vi "Controller Apply Configuration from GUI.vi"(7 "Sync Objects":T9, 8 "error in (no error)":errorcluster, 10 "Configuration Data (GUI to Controller)":T8, 11 "FOFB Configuration":T1={"FOFB Parameters"={"Network"={"FOFB Controller IP"="", "LNLS Control Network IP"="", "LNLS Control Network Power Supplies TCP Port"=0, "LNLS Control Network FOFB Configuration TCP Port"=0, "LNLS Control Network BPMs TCP Port"=0, "Data Server TCP Port"=0, "Monitoring Data TCP Port"=0, "Configuration GUI TCP Port"=0, "Storage Data TCP Port"=0, "Fast Command TCP Port"=0, "TCP Listening Timeout"=0}, "Fast Acquisition"={"Sampling Period"=0, "Data Buffer Size"=0, "Monitoring Period"=0}, "Acquisition Network"=[], "Actuation Network"=[]}, "Number of Acquisition Chassis"=0, "Number of Actuation Chassis"=0, "Number of BPM Readings"=0, "BPM Reading Names"=[], "Selected BPM Readings"=[0, 1, 2, 3, 4, 5, 6, 7, 8, 9, 10, 11, 12, 13, 14, 15, 16, 17, 18, 19, 20, 21, 22, 23, 24, 25, 26, 27, 28, 29, 30, 31, 32, 33, 34, 35, 36, 37, 38, 39, 40, 41, 42, 43, 44, 45, 46, 47, 48, 49], "Number of Correctors"=0, "Corrector Names"=[], "Selected Correctors"=[0, 1, 2, 3, 4, 5, 6, 7, 8, 9, 10, 11, 12, 13, 14, 15, 16, 17, 18, 19, 20, 21, 22, 23, 24, 25, 26, 27, 28, 29, 30, 31, 32, 33, 34, 35, 36, 37, 38, 39, 40, 41, 42, 43, 44, 45, 46, 47, 48, 49], "Reference Orbit"=[], "Response Matrix"=[], "Correction Matrix"=[], "Acquisition Chassis Names"=[], "Actuation Chassis Names"=[], "Acquisition Variables"=[], "Actuation Variables"=[], "PS Matrix Mapping"=[], "Inverse PS Matrix Mapping"=[], "BPM Matrix Mapping"=[], "Inverse BPM Matrix Mapping"=[], "BPM Planes"=[], "Corrector Planes"=[]}) -> (0 "error out":errorcluster, 2 "Configuration Change Acknowledge (Controller to GUI)":T7)   [LabVIEW 2011, in "Controller VIs.lvlib"]
uses:
  Controller VIs.lvlib
  Types Definitions/Type Synchronization Objects.ctl
  Types Definitions/Type Blocking Synchronization Objects.ctl
  Types Definitions/Type Monitoring Data.ctl
  Types Definitions/Type Operation Mode State.ctl
  Types Definitions/Type Diagnostics Data.ctl
  Types Definitions/Type CPU Loads Array.ctl
  Types Definitions/Type CPU Loads.ctl
  Types Definitions/Type Non-blocking Synchronization Objects.ctl
  Types Definitions/Type FOFB Variables.ctl
  Types Definitions/Type Actuation State.ctl
  Types Definitions/Type Configuration Data (GUI to Controller).ctl
  Types Definitions/Type FOFB Parameters.ctl
  Types Definitions/Type Network Configuration.ctl
  Types Definitions/Type FA Configuration.ctl
  Types Definitions/Type Acquisition Network Configuration.ctl
  Types Definitions/Type Actuation Network Configuration.ctl
  Types Definitions/Type Configuration Change Acknowledge (Controller to GUI).ctl
  Types Definitions/Type FOFB Configuration.ctl
  File VIs/File Read Orbit.vi
  File VIs/File Read Matrix.vi
  XML VIs/XML Get Actuation Chassis.vi
  XML VIs/XML Get Acquisition Chassis.vi
  Controller Orbit Correction Matrix Calculation.vi
  File VIs/File Write Matrix.vi
  Type Definitions.lvlib
  XML VIs.lvlib
  File VIs.lvlib
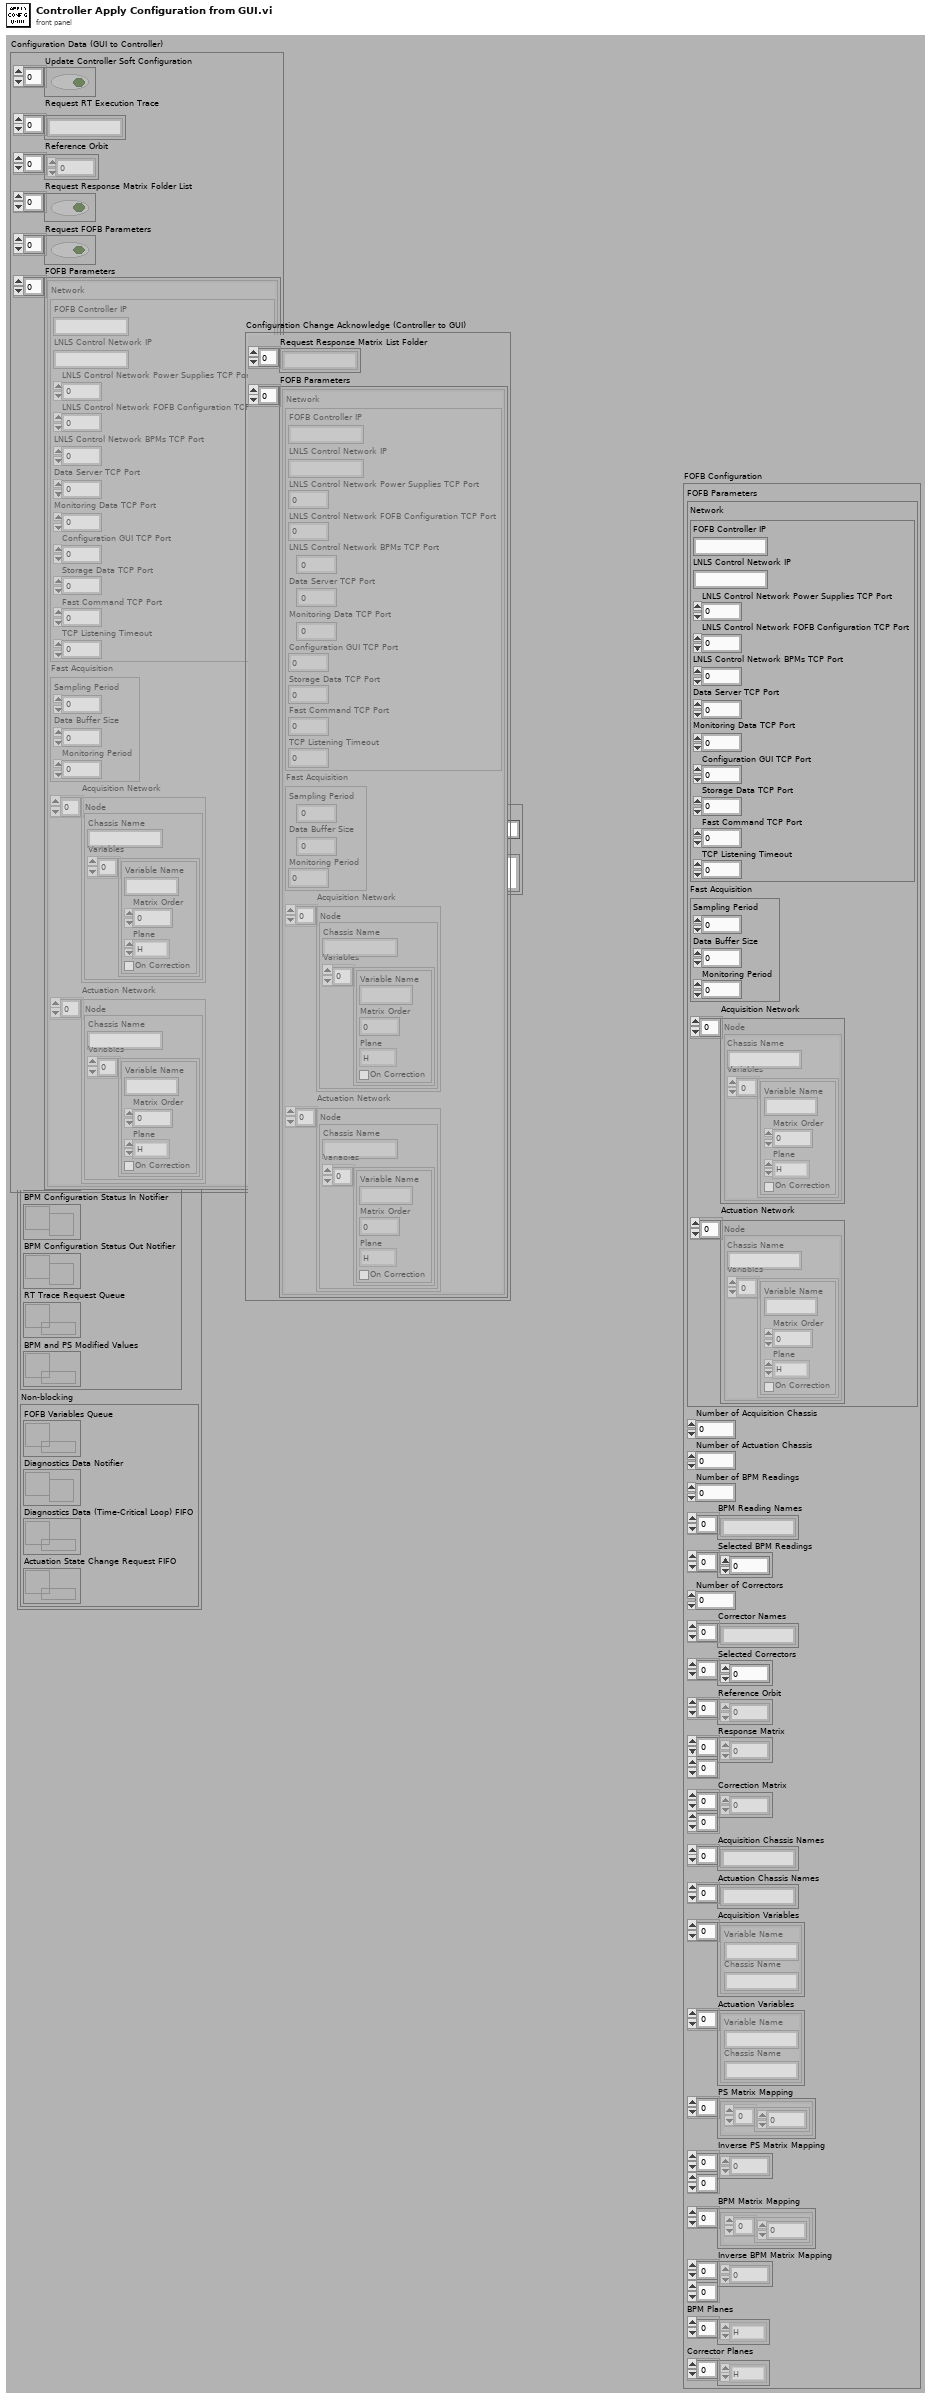
[diagram p1: front panel]
types:
  T1 = typedef "Type Definitions.lvlib/Type FOFB Configuration.ctl" = cluster{"FOFB Parameters":T2, "Number of Acquisition Chassis":i32, "Number of Actuation Chassis":i32, "Number of BPM Readings":i32, "BPM Reading Names":string[], "Selected BPM Readings":u32[], "Number of Correctors":i32, "Corrector Names":string[], "Selected Correctors":u32[], "Reference Orbit":dbl[], "Response Matrix":dbl[][], "Correction Matrix":dbl[][], "Acquisition Chassis Names":string[], "Actuation Chassis Names":string[], "Acquisition Variables":cluster{"Variable Name":string, "Chassis Name":string}[], "Actuation Variables":cluster{"Variable Name":string, "Chassis Name":string}[], "PS Matrix Mapping":cluster{u32[]}[], "Inverse PS Matrix Mapping":u32[][], "BPM Matrix Mapping":cluster{u32[]}[], "Inverse BPM Matrix Mapping":u32[][], "BPM Planes":enum8{"H", "V"}[], "Corrector Planes":enum8{"H", "V"}[]}
  T2 = typedef "Type Definitions.lvlib/Type FOFB Parameters.ctl" = cluster{"Network":T3, "Fast Acquisition":T4, "Acquisition Network":T5, "Actuation Network":T6}
  T3 = typedef "Type Definitions.lvlib/Type Network Configuration.ctl" = cluster{"FOFB Controller IP":string, "LNLS Control Network IP":string, "LNLS Control Network Power Supplies TCP Port":u16, "LNLS Control Network FOFB Configuration TCP Port":u16, "LNLS Control Network BPMs TCP Port":u16, "Data Server TCP Port":u16, "Monitoring Data TCP Port":u16, "Configuration GUI TCP Port":u16, "Storage Data TCP Port":u16, "Fast Command TCP Port":u16, "TCP Listening Timeout":i32}
  T4 = typedef "Type Definitions.lvlib/Type FA Configuration.ctl" = cluster{"Sampling Period":u32, "Data Buffer Size":u32, "Monitoring Period":u32}
  T5 = typedef "Type Definitions.lvlib/Type Acquisition Network Configuration.ctl" = cluster{"Chassis Name":string, "Variables":cluster{"Variable Name":string, "Matrix Order":u32, "Plane":enum8{"H", "V"}, "On Correction":bool}[]}[]
  T6 = typedef "Type Definitions.lvlib/Type Actuation Network Configuration.ctl" = cluster{"Chassis Name":string, "Variables":cluster{"Variable Name":string, "Matrix Order":u32, "Plane":enum8{"H", "V"}, "On Correction":bool}[]}[]
  T7 = typedef "Type Definitions.lvlib/Type Configuration Change Acknowledge (Controller to GUI).ctl" = cluster{"Request Response Matrix List Folder":string[], "FOFB Parameters":T2[]}
  T8 = typedef "Type Definitions.lvlib/Type Configuration Data (GUI to Controller).ctl" = cluster{"Update Controller Soft Configuration":bool[], "Request RT Execution Trace":string[], "Reference Orbit":dbl[], "Request Response Matrix Folder List":bool[], "Request FOFB Parameters":bool[], "FOFB Parameters":T2[]}
  T9 = typedef "Type Definitions.lvlib/Type Synchronization Objects.ctl" = cluster{"Blocking":T10, "Non-blocking":T11}
  T10 = typedef "Type Definitions.lvlib/Type Blocking Synchronization Objects.ctl" = cluster{"Monitoring Data Notifier":refnum<notifier>, "Storage Data FIFO":refnum<queue>, "Operation Mode Change Request FIFO":refnum<k33>, "Monitoring BPM and PS Data FIFO":refnum<k33>, "FA BPM and PS Data FIFO":refnum<k33>, "PS Manual Setpoints FIFO":refnum<k33>, "FOFB Controller Errors FIFO ":refnum<k33>, "FOFB Status In Notifier":refnum<notifier>, "FOFB Status Out Notifier":refnum<notifier>, "PS Configuration Status In Notifier":refnum<notifier>, "PS Configuration Status Out Notifier":refnum<notifier>, "BPM Configuration Status In Notifier":refnum<notifier>, "BPM Configuration Status Out Notifier":refnum<notifier>, "RT Trace Request Queue":refnum<queue>, "BPM and PS Modified Values":refnum<k33>}
  T11 = typedef "Type Definitions.lvlib/Type Non-blocking Synchronization Objects.ctl" = cluster{"FOFB Variables Queue":refnum<queue>, "Diagnostics Data Notifier":refnum<notifier>, "Diagnostics Data (Time-Critical Loop) FIFO":refnum<k33>, "Actuation State Change Request FIFO":refnum<k33>}
  T12 = typedef "Type Definitions.lvlib/Type FOFB Variables.ctl" = cluster{"Reference Orbit":dbl[], "Response Matrix":dbl[][], "Correction Matrix":dbl[][], "Selected BPM Readings":u32[], "Selected Correctors":u32[], "BPM Planes":enum8{"H", "V"}[], "Corrector Planes":enum8{"H", "V"}[], "Fast Command Enabled":bool, "Horizontal Gain":dbl, "Vertical Gain":dbl}
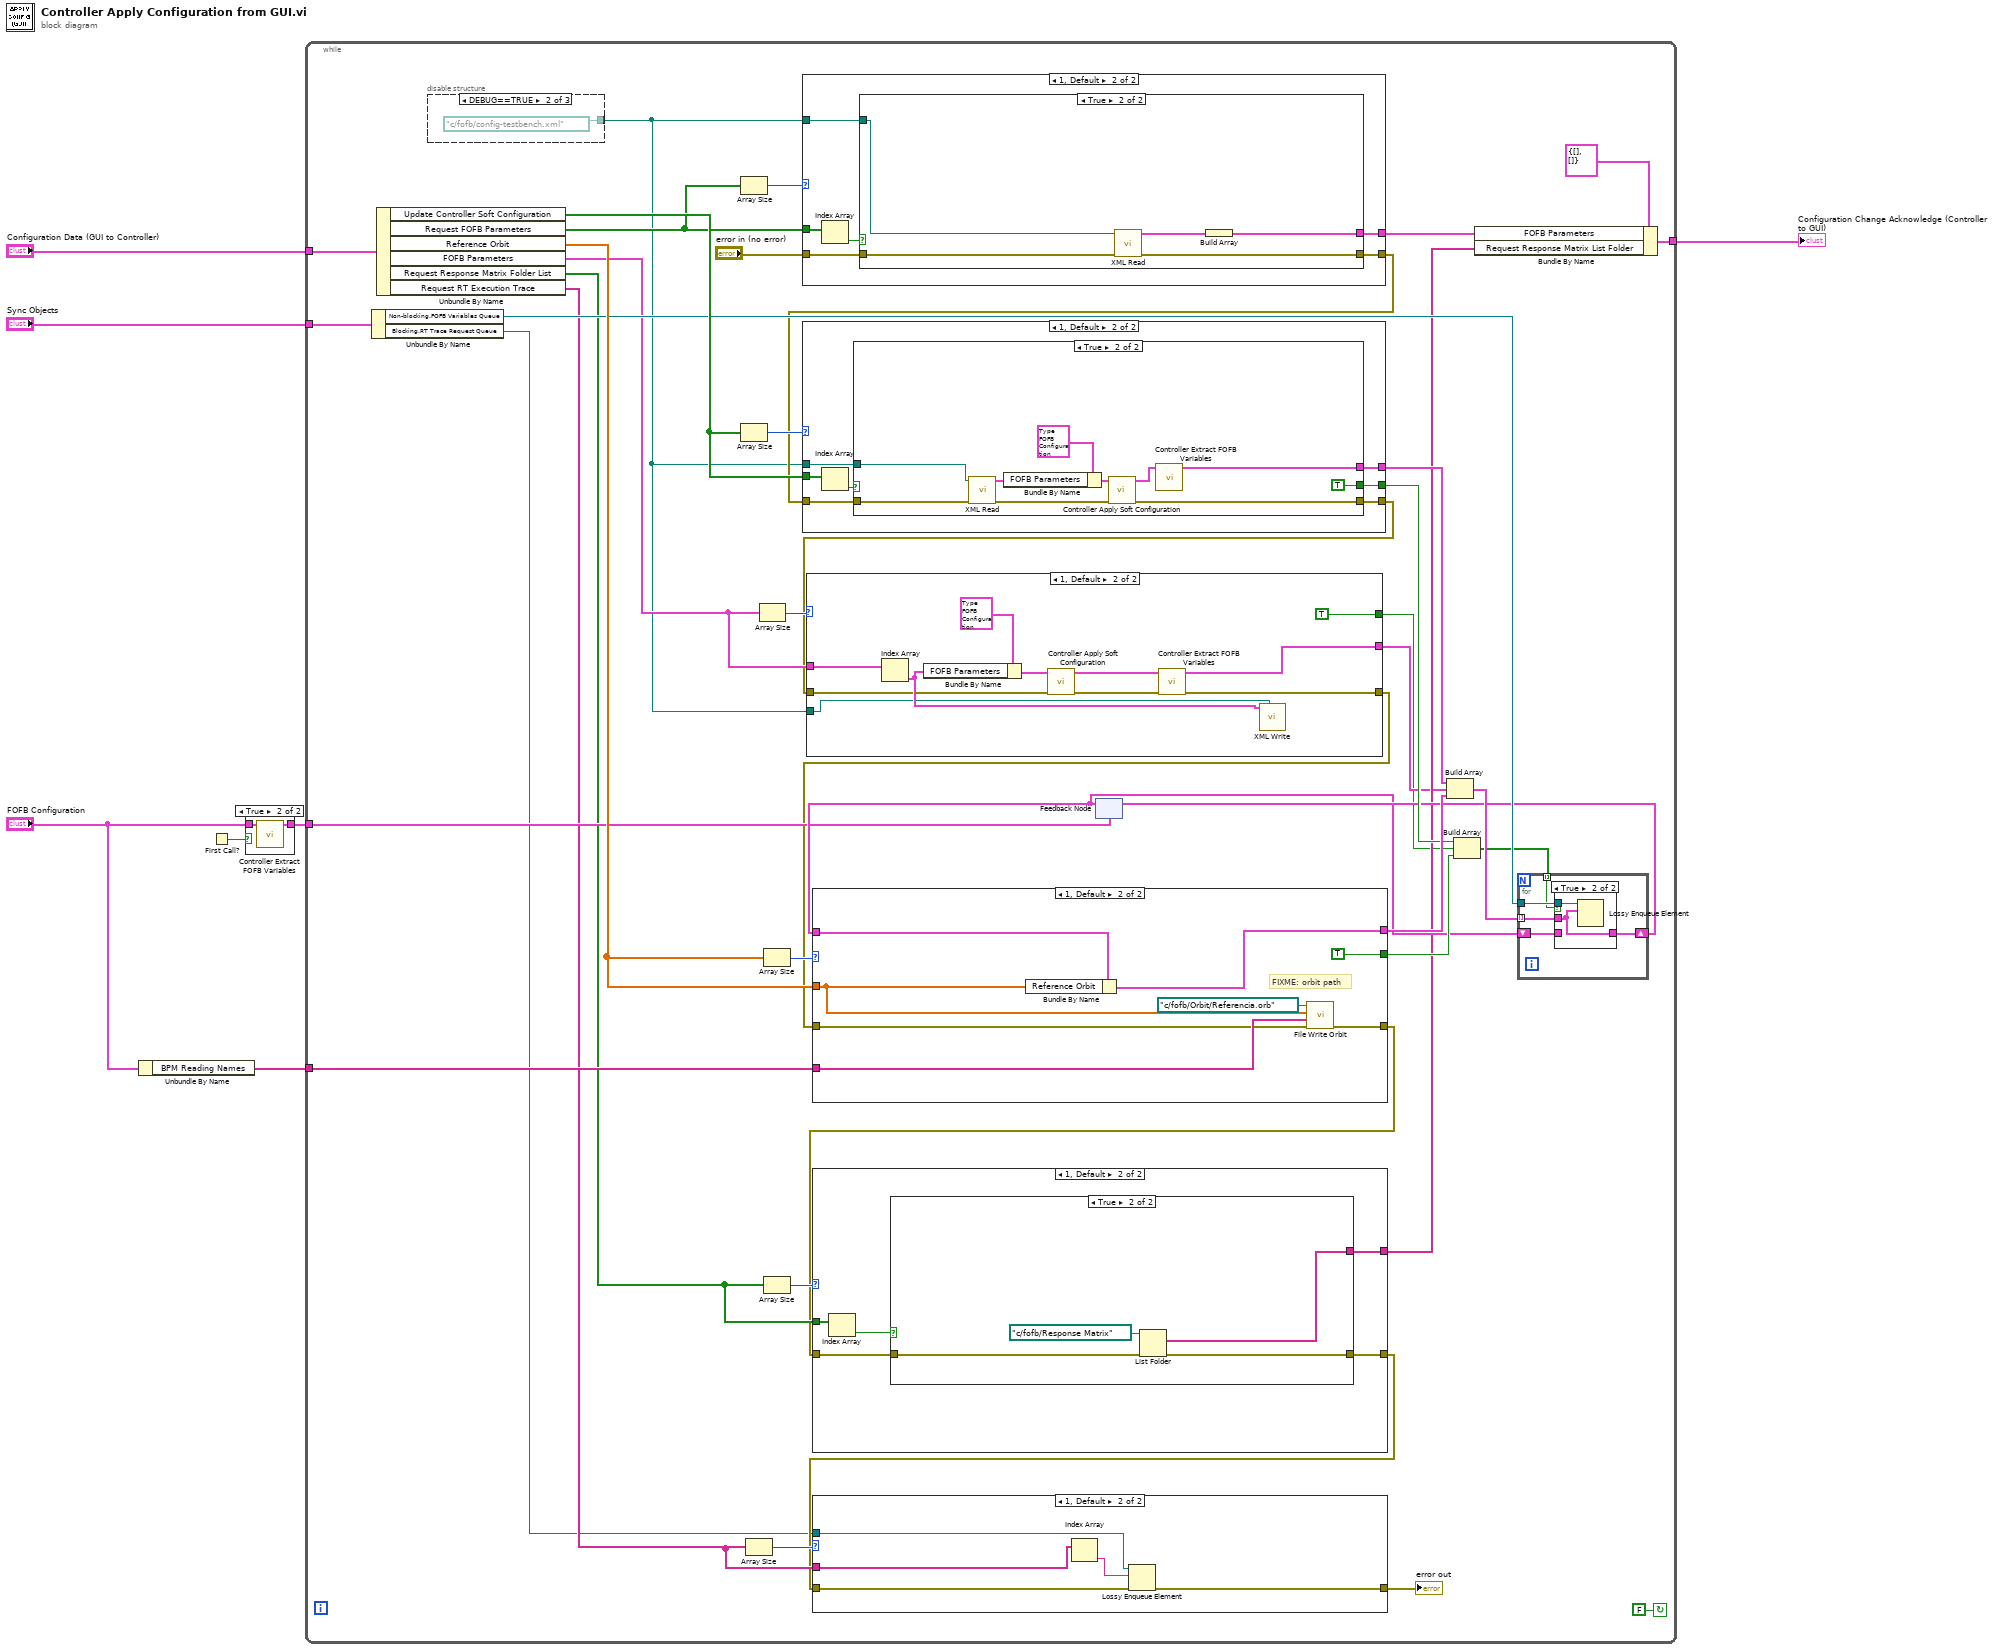
[diagram p0: block diagram]
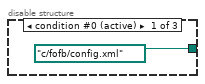
[diagram p4: hidden frame]
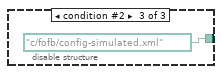
[diagram p5: hidden frame]
diagram:
  n1 = Unbundle By Name("FOFB Configuration") -> ("BPM Reading Names"=w1:string[])
  n2 = First Call?() -> (First Call?: T/F=w4:bool)
  n3 = case shown="True" w4 {
    tunnel: "FOFB Configuration" -> [_ w9]
    tunnel: [_ w8] -> w3
    frame False {
    }
    frame True {
      n4 = call "Controller Extract FOFB Variables.vi"("FOFB Configuration"=w9) -> ("FOFB Variables"=w8:T12)  [unwired: 9 in, 1 out]
    }
  }
  n5 = while {
    tunnel: "Sync Objects" -> [w50]
    tunnel: "Configuration Data (GUI to Controller)" -> [w49]
    tunnel: [w40] -> w5
    tunnel: w3 -> [w28]
    tunnel: w1 -> [w27]
    stop <- FALSE continue-if-true
    n6 = Unbundle By Name(w50) -> ("Non-blocking.FOFB Variables Queue"=w39:refnum<queue>, "Blocking.RT Trace Request Queue"=w17:refnum<queue>)
    n7 = Unbundle By Name(w49) -> ("Update Controller Soft Configuration"=w46:bool[], "Request FOFB Parameters"=w44:bool[], "Reference Orbit"=w41:dbl[], "FOFB Parameters"=w15:T2[], "Request Response Matrix Folder List"=w25:bool[], "Request RT Execution Trace"=w20:string[])
    n8 = disable-structure shown="DEBUG==TRUE" {
      disable-tunnel: [path "c:/fofb/config.xml" ("Configuration File Path") path "c:/fofb/config-testbench.xml" ("Configuration File Path") path "c:/fofb/config-simulated.xml" ("Configuration File Path")] -> w13
      frame condition #0 (active) {
      }
      frame condition #1 {
      }
      frame condition #2 {
      }
    }
    n9 = Array Size(array=w44) -> (size(s)=w45:i32)
    n10 = Array Size(array=w46) -> (size(s)=w47:i32)
    n11 = Array Size(array=w20) -> (size(s)=w21:i32)
    n12 = Array Size(array=w15) -> (size(s)=w16:i32)
    n13 = Array Size(array=w41) -> (size(s)=w42:i32)
    n14 = Array Size(array=w25) -> (size(s)=w26:i32)
    n15 = case shown="1, Default" w45 {
      tunnel: w44 -> [_ w107]
      tunnel: "error in (no error)" -> [w101 w105]
      tunnel: [w101 w104] -> w38
      tunnel: [_ w103] -> w43
      tunnel: w13 -> [_ w102]
      frame 0 {
      }
      frame 1, Default {
        n16 = Index Array(array=w107) -> (element=w106:bool)  [unwired: 1 in]
        n17 = case shown="True" w106 {
          tunnel: w105 -> [w108 w113]
          tunnel: [w108 w112] -> w104
          tunnel: [_ w111] -> w103
          tunnel: w102 -> [_ w109]
          frame False {
          }
          frame True {
            n18 = call "XML Read.vi"("error in"=w113, "XML File Path In"=w109) -> ("error out"=w112:errorcluster, "FOFB Parameters"=w110:T2)  [unwired: 8 in]
            n19 = Build Array(w110) -> (w111:T2[])
          }
        }
      }
    }
    n20 = case shown="1, Default" w47 {
      tunnel: w46 -> [_ w121]
      tunnel: w38 -> [w114 w119]
      tunnel: [w114 w117] -> w11
      tunnel: [_ w118] -> w37
      tunnel: [_ w116] -> w35
      tunnel: w13 -> [_ w115]
      frame 0 {
      }
      frame 1, Default {
        n21 = Index Array(array=w121) -> (element=w120:bool)  [unwired: 1 in]
        n22 = case shown="True" w120 {
          tunnel: w119 -> [w122 w129]
          tunnel: [w122 w126] -> w117
          tunnel: [_ w125] -> w118
          tunnel: [_ TRUE] -> w116
          tunnel: w115 -> [_ w123]
          frame False {
          }
          frame True {
            n23 = call "XML Read.vi"("error in"=w129, "XML File Path In"=w123) -> ("error out"=w132:errorcluster, "FOFB Parameters"=w130:T2)  [unwired: 8 in]
            n24 = Bundle By Name(cluster=T1 {"FOFB Parameters"={"Network"={"FOFB Controller IP"="", "LNLS Control Network IP"="", "LNLS Control Network Power Supplies TCP Port"=0, "LNLS Control Network FOFB Configuration TCP Port"=0, "LNLS Control Network BPMs TCP Port"=0, "Data Server TCP Port"=0, "Monitoring Data TCP Port"=0, "Configuration GUI TCP Port"=0, "Storage Data TCP Port"=0, "Fast Command TCP Port"=0, "TCP Listening Timeout"=0}, "Fast Acquisition"={"Sampling Period"=0, "Data Buffer Size"=0, "Monitoring Period"=0}, "Acquisition Network"=[], "Actuation Network"=[]}, "Number of Acquisition Chassis"=0, "Number of Actuation Chassis"=0, "Number of BPM Readings"=0, "BPM Reading Names"=[], "Selected BPM Readings"=[], "Number of Correctors"=0, "Corrector Names"=[], "Selected Correctors"=[], "Reference Orbit"=[], "Response Matrix"=[], "Correction Matrix"=[], "Acquisition Chassis Names"=[], "Actuation Chassis Names"=[], "Acquisition Variables"=[], "Actuation Variables"=[], "PS Matrix Mapping"=[], "Inverse PS Matrix Mapping"=[], "BPM Matrix Mapping"=[], "Inverse BPM Matrix Mapping"=[], "BPM Planes"=[], "Corrector Planes"=[]}, "FOFB Parameters"=w130) -> (w131:T1)
            n25 = call "Controller Apply Soft Configuration.vi"("error in (no error)"=w132, "FOFB Configuration"=w131) -> ("error out"=w126:errorcluster, "FOFB Configuration"=w128:T1)  [unwired: 8 in]
            n26 = call "Controller Extract FOFB Variables.vi"("FOFB Configuration"=w128) -> ("FOFB Variables"=w125:T12)  [unwired: 9 in, 1 out]
          }
        }
      }
    }
    n27 = case shown="1, Default" w16 {
      tunnel: w15 -> [_ w62]
      tunnel: [_ w58] -> w14
      tunnel: w13 -> [_ w56]
      tunnel: [_ TRUE] -> w12
      tunnel: w11 -> [w51 w54]
      tunnel: [w51 w52] -> w10
      frame 0 {
      }
      frame 1, Default {
        n28 = Index Array(array=w62) -> (element=w57:T2)  [unwired: 1 in]
        n29 = Bundle By Name(cluster=T1 {"FOFB Parameters"={"Network"={"FOFB Controller IP"="", "LNLS Control Network IP"="", "LNLS Control Network Power Supplies TCP Port"=0, "LNLS Control Network FOFB Configuration TCP Port"=0, "LNLS Control Network BPMs TCP Port"=0, "Data Server TCP Port"=0, "Monitoring Data TCP Port"=0, "Configuration GUI TCP Port"=0, "Storage Data TCP Port"=0, "Fast Command TCP Port"=0, "TCP Listening Timeout"=0}, "Fast Acquisition"={"Sampling Period"=0, "Data Buffer Size"=0, "Monitoring Period"=0}, "Acquisition Network"=[], "Actuation Network"=[]}, "Number of Acquisition Chassis"=0, "Number of Actuation Chassis"=0, "Number of BPM Readings"=0, "BPM Reading Names"=[], "Selected BPM Readings"=[], "Number of Correctors"=0, "Corrector Names"=[], "Selected Correctors"=[], "Reference Orbit"=[], "Response Matrix"=[], "Correction Matrix"=[], "Acquisition Chassis Names"=[], "Actuation Chassis Names"=[], "Acquisition Variables"=[], "Actuation Variables"=[], "PS Matrix Mapping"=[], "Inverse PS Matrix Mapping"=[], "BPM Matrix Mapping"=[], "Inverse BPM Matrix Mapping"=[], "BPM Planes"=[], "Corrector Planes"=[]}, "FOFB Parameters"=w57) -> (w60:T1)
        n30 = call "Controller Apply Soft Configuration.vi"("error in (no error)"=w54, "FOFB Configuration"=w60) -> ("error out"=w53:errorcluster, "FOFB Configuration"=w59:T1)  [unwired: 8 in]
        n31 = call "Controller Extract FOFB Variables.vi"("error in (no error)"=w53, "FOFB Configuration"=w59) -> ("error out"=w52:errorcluster, "FOFB Variables"=w58:T12)  [unwired: 8 in]
        n32 = call "XML Write.vi"("XML File Path Write"=w56, "FOFB Parameters"=w57) -> ()  [unwired: 8 in, 2 out]
      }
    }
    n33 = feedback #1(w28) -> (w30:T12)
    n34 = case shown="1, Default" w42 {
      tunnel: w41 -> [_ w97]
      tunnel: w10 -> [w92 w95]
      tunnel: [w92 w94] -> w24
      tunnel: w30 -> [w91 w100]
      tunnel: [_ TRUE] -> w34
      tunnel: [w91 w98] -> w36
      tunnel: w27 -> [_ w96]
      frame 0 {
      }
      frame 1, Default {
        # "FIXME: orbit path"
        n35 = Bundle By Name(cluster=w100, "Reference Orbit"=w97) -> (w98:T12)
        n36 = call "File Write Orbit.vi"("error in (no error)"=w95, "BPM Reading Names"=w96, "Orbit"=w97, "file path (dialog if empty)"=path "c:/fofb/Orbit/Referencia.orb") -> ("error out"=w94:errorcluster)  [unwired: 6 in]
      }
    }
    n37 = case shown="1, Default" w26 {
      tunnel: w24 -> [w72 w75]
      tunnel: [w72 w74] -> w19
      tunnel: w25 -> [_ w77]
      tunnel: [_ w73] -> w22
      frame 0 {
      }
      frame 1, Default {
        n38 = Index Array(array=w77) -> (element=w76:bool)  [unwired: 1 in]
        n39 = case shown="True" w76 {
          tunnel: w75 -> [w78 w81]
          tunnel: [w78 w80] -> w74
          tunnel: [_ w79] -> w73
          frame False {
          }
          frame True {
            n40 = List Folder(path=path "c:/fofb/Response Matrix", error in=w81) -> (filenames=w79:string[], error out=w80:errorcluster)  [unwired: 2 in, 2 out]
          }
        }
      }
    }
    n41 = case shown="1, Default" w21 {
      tunnel: w20 -> [_ w71]
      tunnel: w17 -> [_ w69]
      tunnel: w19 -> [w66 w68]
      tunnel: [w66 w67] -> w18
      frame 0 {
      }
      frame 1, Default {
        n42 = Index Array(array=w71) -> (element=w70:string)  [unwired: 1 in]
        n43 = Lossy Enqueue Element(queue=w69, element=w70, error in (no error)=w68) -> (error out=w67:errorcluster)  [unwired: 3 out]
      }
    }
    "error out" <- w18
    n44 = Build Array(w37, w14, w36) -> (w33:T12[])
    n45 = Build Array(w35, w12, w34) -> (w32:bool[])
    n46 = Bundle By Name(cluster=T7 {"Request Response Matrix List Folder"=[], "FOFB Parameters"=[]} ("Configuration Change Acknowledge (Controller to GUI)"), "FOFB Parameters"=w43, "Request Response Matrix List Folder"=w22) -> (w40:T7)
    n47 = for {
      tunnel: w39 -> [w87]
      tunnel: w33 -> [w85] mode=indexing
      tunnel: w32 -> [w86] mode=indexing
      shift-right: [w84] -> w31
      shift-left: w30 -> [w83]
      n48 = case shown="True" w86 {
        tunnel: w87 -> [_ w90]
        tunnel: w85 -> [_ w89]
        tunnel: [w88 w89] -> w84
        tunnel: w83 -> [w88 _]
        frame False {
        }
        frame True {
          n49 = Lossy Enqueue Element(queue=w90, element=w89) -> ()  [unwired: 1 in, 4 out]
        }
      }
    }
    n50 = feedback-in #1(w31) -> ()
  }
  "Configuration Change Acknowledge (Controller to GUI)" <- w5
